vi "RandomInsertionBenchmark.vi"() -> ()   [LabVIEW 2009]
uses:
  ImpSelectionEnum.ctl
  source/Lists/ListImp/ListImp.lvclass
  source/Lists.Implementations/BufferedArray/BufferedArray.lvclass
  source/Lists.Interfaces/StringList/StringList.lvclass
  <vilib>/Analysis/NI_AALBase.lvlib
panel:
  out "Histogram Graph":T1(graph)
  in  "Number of Elements":i32
  in  "Implementation":T2
  out "Buffered Array List Imp":u32
  out "Default List Imp":u32
  out "error out":errorcluster
  # "Random Insertion"
  # "50,000 elements is sufficient to see the difference in time for each of the implementations."
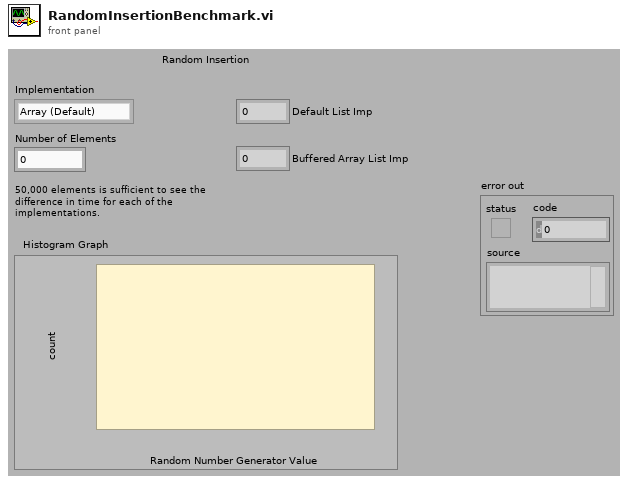
[diagram p1: front panel]
types:
  T1 = cluster{"X Values":dbl[], "Histogram: h(x)":i32[]}
  T2 = typedef "ImpSelectionEnum.ctl" = enum16{"Array (Default)", "Buffered Array"}
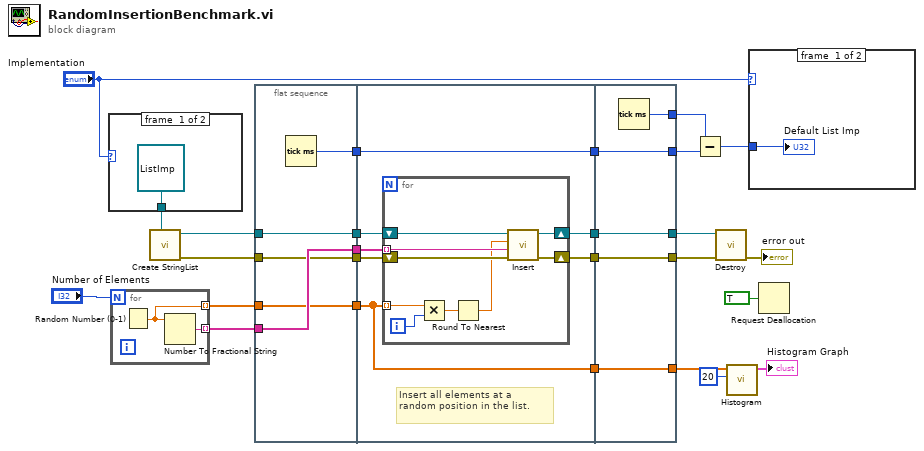
[diagram p0: block diagram]
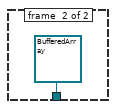
[diagram p2: hidden frame]
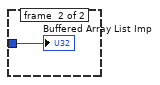
[diagram p3: hidden frame]
diagram:
  n1 = case shown="\"Array (Default)\", Default" "Implementation" {
    tunnel: [refnum<class "ListImp.lvclass"> refnum ("LapDog.Collections.v0.Lists.lvlib:ListImp.lvclass") refnum<class "BufferedArray.lvclass"> refnum ("LapDog.Collections.v0.Lists.Implementations.lvlib:BufferedArray.lvclass")] -> w22
    frame #0 {
    }
    frame #1 {
    }
  }
  n2 = for {
    N: "Number of Elements" -> [_]
    tunnel: [w30] -> w25 mode=indexing
    tunnel: [w29] -> w7 mode=indexing
    n3 = Random Number (0-1)() -> (number: 0 to 1=w29:dbl)
    n4 = Number To Fractional String(number=w29) -> (F-format string=w30:string)  [unwired: 3 in]
  }
  n5 = call "Create StringList.vi"("List Implementation (Array)"=w22) -> ("error out"=w18:errorcluster, "StringList out"=w20:refnum<class "StringList.lvclass">)  [unwired: 9 in]
  n6 = flat-sequence {
    tunnel: w25 -> [w35]
    tunnel: [w35] -> w24
    tunnel: [w34] -> w23
    tunnel: [w33] -> w21
    tunnel: w20 -> [w33]
    tunnel: [w32] -> w19
    tunnel: w18 -> [w32]
    tunnel: [w31] -> w8
    tunnel: w7 -> [w31]
    tunnel: w24 -> [w42]
    tunnel: w23 -> [w37]
    tunnel: w21 -> [w41]
    tunnel: w19 -> [w40]
    tunnel: [w39] -> w17
    tunnel: [w38] -> w16
    tunnel: [w37] -> w15
    tunnel: w8 -> [w36]
    tunnel: [w36] -> w6
    tunnel: [w55] -> w2
    tunnel: [w56] -> w1
    tunnel: w17 -> [w56]
    tunnel: w16 -> [w55]
    tunnel: w15 -> [w53]
    tunnel: [w54] -> w14
    tunnel: [w53] -> w13
    tunnel: [w52] -> w5
    tunnel: w6 -> [w52]
    frame #0 {
      n7 = Tick Count (ms)() -> (millisecond timer value=w34:u32)
    }
    frame #1 {
      # "Insert all elements at a random position in the list."
      n8 = for {
        shift-right: [w50] -> w39
        shift-left: w41 -> [w51]
        tunnel: w42 -> [w49] mode=indexing
        shift-right: [w47] -> w38
        shift-left: w40 -> [w48]
        tunnel: w36 -> [w46] mode=indexing
        i -> [w45]
        n9 = Multiply(x=w46, y=w45) -> (x*y=w44:dbl)
        n10 = Round To Nearest(number=w44) -> (nearest integer value=w43:dbl)
        n11 = call-dynamic "Insert.vi"("error in (no error)"=w48, "String"=w49, "Index"=w43, "StringList in"=w51) -> ("error out"=w47:errorcluster, "StringList out"=w50:refnum<class "StringList.lvclass">)  [unwired: 6 in]
      }
    }
    frame #2 {
      n12 = Tick Count (ms)() -> (millisecond timer value=w54:u32)
    }
  }
  n13 = Subtract(x=w14, y=w13) -> (x-y=w11:u32)
  n14 = call-dynamic "Destroy.vi"("error in (no error)"=w2, "StringList in"=w1) -> ("error out"=→"error out":errorcluster)  [unwired: 9 in]
  n15 = call <vilib>:"Histogram.vi"("intervals"=20, "X"=w5) -> ("Histogram Graph"=→"Histogram Graph":T1)  [unwired: 6 in, 3 out]
  n16 = case shown="\"Array (Default)\", Default" "Implementation" {
    tunnel: w11 -> [w57 w58]
    frame #0 {
      "Default List Imp" <- w57
    }
    frame #1 {
      "Buffered Array List Imp" <- w58
    }
  }
  n17 = Request Deallocation(TRUE ("flag")) -> ()
